vi "test Option as Flag Just Has Set.vi"(8 "error in (no error)":errorcluster, 11 "TestCase in":refnum<class "Options Parsing Tests.lvclass">) -> (0 "error out":errorcluster, 3 "TestCase out":refnum<class "Options Parsing Tests.lvclass">)   [LabVIEW 2015, in "Options Parsing Tests.lvclass"]
uses:
  Options Parsing Tests.lvclass
  Argument Parser/Option Class/Option Configuration.ctl
  Argument Parser/Option Class/Argument Type.ctl
  <vilib>/addons/_JKI Toolkits/VI Tester/TestCase.llb/TestCase.lvclass
  Argument Parser/Option Set Class/Option Set.lvclass
  Argument Parser/Option Class/Option.lvclass
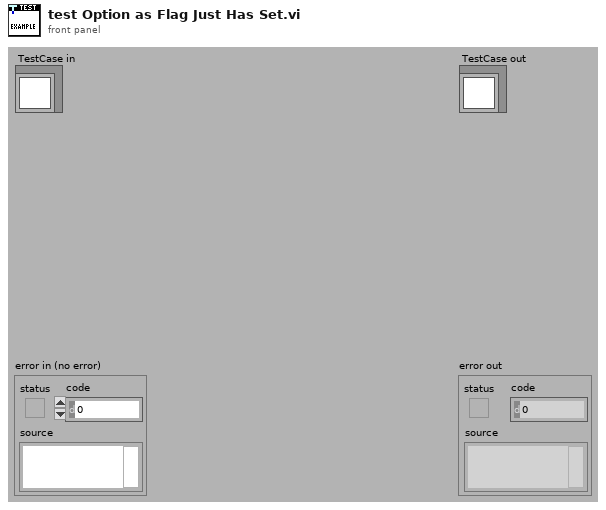
[diagram p1: front panel]
types:
  T1 = typedef "Option Parser.lvlib/Option.lvclass/Option Configuration.ctl" = cluster{"Option Type":T2, "Option Labels":string[], "Key":string, "Description":string, "Required":bool, "Default Value":string}
  T2 = typedef "Option Parser.lvlib/Option.lvclass/Argument Type.ctl" = enum16{"flag", "value"}
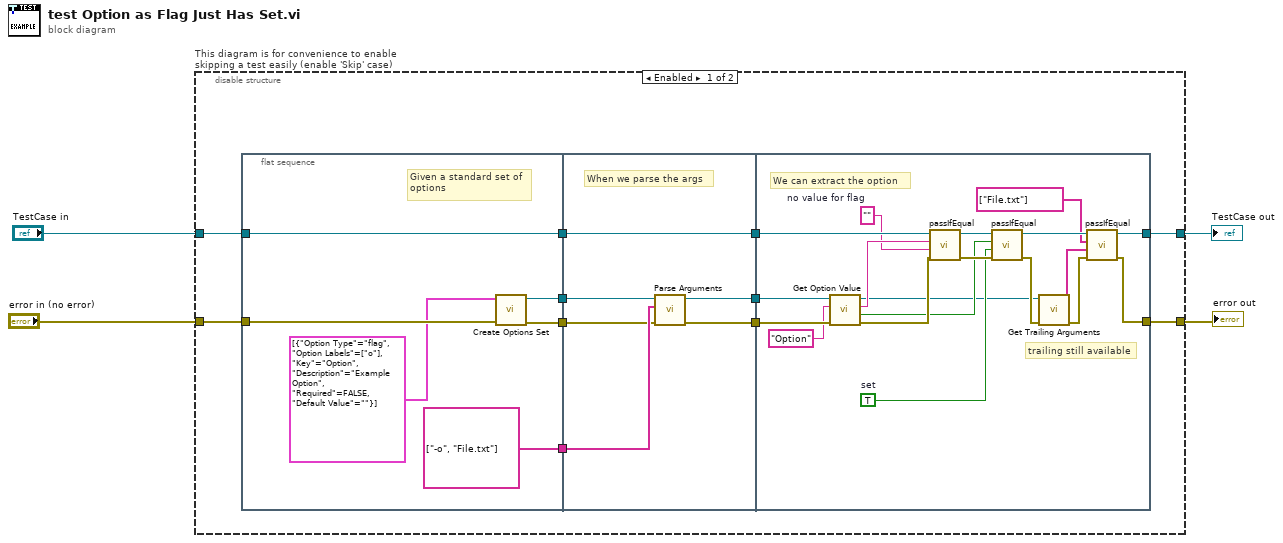
[diagram p0: block diagram]
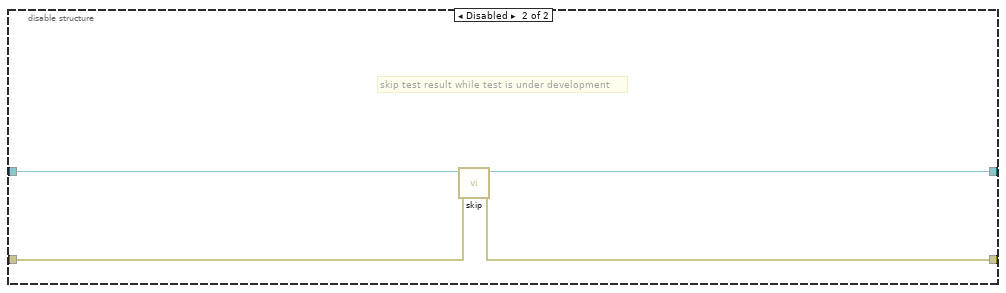
[diagram p2: hidden frame]
diagram:
  n1 = disable-structure "This diagram is for convenience to enable skipping a test easily (enable 'Skip' case)" shown="Enabled" {
    disable-tunnel: "TestCase in" -> [w7 w50]
    disable-tunnel: [w6 w48] -> w1
    disable-tunnel: [w5 w49] -> w3
    disable-tunnel: "error in (no error)" -> [w14 w47]
    frame Enabled {
      n2 = flat-sequence {
        tunnel: [string[] ["-o", "File.txt"]] -> w15
        tunnel: w14 -> [w20]
        tunnel: [w19] -> w13
        tunnel: [w18] -> w12
        tunnel: [w17] -> w8
        tunnel: w7 -> [w17]
        tunnel: w15 -> [w27]
        tunnel: w13 -> [w26]
        tunnel: w12 -> [w25]
        tunnel: [w24] -> w11
        tunnel: [w23] -> w10
        tunnel: [w22] -> w9
        tunnel: w8 -> [w22]
        tunnel: w11 -> [w46]
        tunnel: w10 -> [w45]
        tunnel: w9 -> [w43]
        tunnel: [w32] -> w6
        tunnel: [w34] -> w5
        frame #0 {
          # "Given a standard set of\noptions"
          n3 = call "Create Options Set.vi"("error in (no error)"=w20, "Options"=T1[] [{"Option Type"=enum."flag", "Option Labels"=["o"], "Key"="Option", "Description"="Example Option", "Required"=FALSE, "Default Value"=""}]) -> ("error out"=w19:errorcluster, "Option Set out"=w18:refnum<class "Option Set.lvclass">)  [unwired: 8 in]
        }
        frame #1 {
          # "When we parse the args"
          n4 = call "Parse Arguments.vi"("error in (no error)"=w26, "Arguments"=w27, "Option Set in"=w25) -> ("error out"=w23:errorcluster, "Option Set out"=w24:refnum<class "Option Set.lvclass">)  [unwired: 5 in, 2 out]
        }
        frame #2 {
          w36 = TRUE  # set
          w35 = ""  # no value for flag
          # "trailing still available"
          # "We can extract the option"
          n5 = call "Get Option Value.vi"("error in (no error)"=w45, "Option Key"="Option", "Option Set in"=w46) -> ("error out"=w42:errorcluster, "Set"=w37:bool, "Value"=w40:string, "Option Set out"=w30:refnum<class "Option Set.lvclass">)  [unwired: 5 in]
          n6 = call-dynamic "passIfEqual.vi"("error in (no error)"=w42, "y"=w35, "x"=w40, "TestCase in"=w43) -> ("error out"=w41:errorcluster, "TestCase out"=w38:refnum<class "Options Parsing Tests.lvclass">)  [unwired: 6 in]
          n7 = call-dynamic "passIfEqual.vi"("error in (no error)"=w41, "y"=w36, "x"=w37, "TestCase in"=w38) -> ("error out"=w39:errorcluster, "TestCase out"=w33:refnum<class "Options Parsing Tests.lvclass">)  [unwired: 6 in]
          n8 = call "Get Trailing Arguments.vi"("error in (no error)"=w39, "Option Set in"=w30) -> ("error out"=w31:errorcluster, "Arguments"=w29:string[])  [unwired: 7 in, 1 out]
          n9 = call-dynamic "passIfEqual.vi"("error in (no error)"=w31, "y"=w29, "x"=string[] ["File.txt"] ("Arguments"), "TestCase in"=w33) -> ("error out"=w34:errorcluster, "TestCase out"=w32:refnum<class "Options Parsing Tests.lvclass">)  [unwired: 6 in]
        }
      }
    }
    frame Disabled {
      # "skip test result while test is under development"
      n10 = call <vilib>:"skip.vi"("error in (no error)"=w47, "TestCase in"=w50) -> ("error out"=w49:errorcluster, "TestCase out"=w48:refnum<class "Options Parsing Tests.lvclass">)  [unwired: 8 in]
    }
  }
  "error out" <- w3
  "TestCase out" <- w1
